vi "CGTdaq dev V4.vi"() -> ()   [LabVIEW 2023]
panel:
  in  "?":bool
  in  "?":bool
  in  "Path":path
  in  "File extension":string
  in  "Filename":string
  out "?":timestamp
  in  "stop":bool
  in  "?":bool
  in  "?":bool
  in  "?":T1(tab)
  in  "Plotted Port":dbl
  out "?":dbl(graph)
  in  "Input Val":dbl
  out "LabJack Error":errorcluster
  out "Error Message":string
  in  "Scan Rate (Hz)":dbl=10.0 format="%.3f"
  out "# Scans Read":i32
  out "Actual Scan Rate (Hz)":dbl format="%.3f"
  out "UD Backlog [%]":dbl format="%.2f"
  in  "Scans To Read Per Iteration":dbl=1.0 format="%.3f"
  out "Comm Backlog [%]":dbl format="%.2f"
  in  "Delay [ms]":u32
  in  "Res Index":dbl
  out "Full filepath":string
  out "A5 Scaled":dbl(graph)
  out "A4 Scaled":dbl(graph)
  out "A3 Scaled":dbl(graph)
  out "A2 Scaled":dbl(graph)
  out "A1 Scaled":dbl(graph)
  out "A0 Scaled":dbl(graph)
  out "A1":dbl
  out "A1_Voltage":dbl
  out "A1_Instrumentlabel":string
  out "A2 X1 2":dbl caption="A0 X1"
  out "A2 X2 2":dbl caption="A0 X2"
  out "A2 X3 2":dbl caption="A0 X3"
  out "A2 B 2":dbl caption="A0 B"
  out "A2 scaled 2":dbl caption="A0 scaled"
  out "A1_Instrumentlabel 2":string
  out "A1_Voltage 3":dbl
  out "A1 2":dbl
  out "A2 X1 3":dbl caption="A0 X1"
  out "A2 X2 3":dbl caption="A0 X2"
  out "A2 X3 3":dbl caption="A0 X3"
  out "A2 B 3":dbl caption="A0 B"
  out "A2 scaled 3":dbl caption="A0 scaled"
  out "A2 scaled 4":dbl caption="A0 scaled"
  out "A1_Instrumentlabel 3":string
  out "A2 X1 4":dbl caption="A0 X1"
  out "A2 X2 4":dbl caption="A0 X2"
  out "A2 X3 4":dbl caption="A0 X3"
  out "A2 B 4":dbl caption="A0 B"
  out "A1_Voltage 2":dbl
  out "A1 3":dbl
  out "A1_Instrumentlabel 4":string
  out "A1 4":dbl
  out "A1_Voltage 4":dbl
  out "A2 scaled 5":dbl caption="A0 scaled"
  out "A2 X2 5":dbl caption="A0 X2"
  out "A2 X3 5":dbl caption="A0 X3"
  out "A2 B 5":dbl caption="A0 B"
  out "A2 X1 5":dbl caption="A0 X1"
  out "A1_Instrumentlabel 5":string
  out "A1 5":dbl
  out "A1_Voltage 5":dbl
  out "A2 X1 6":dbl caption="A0 X1"
  out "A2 X2 6":dbl caption="A0 X2"
  out "A2 X3 6":dbl caption="A0 X3"
  out "A2 B 6":dbl caption="A0 B"
  out "A2 scaled 6":dbl caption="A0 scaled"
  out "A1_Instrumentlabel 6":string
  out "A1 6":dbl
  out "A1_Voltage 6":dbl
  out "A2 X1 7":dbl caption="A0 X1"
  out "A2 X2 7":dbl caption="A0 X2"
  out "A2 X3 7":dbl caption="A0 X3"
  out "A2 B 7":dbl caption="A0 B"
  out "A2 scaled 7":dbl caption="A0 scaled"
  out "A1_Instrumentlabel 7":string
  out "A1 7":dbl
  out "A1_Voltage 7":dbl
  out "A2 scaled 8":dbl caption="A0 scaled"
  out "A2 X2 8":dbl caption="A0 X2"
  out "A2 X1 8":dbl caption="A0 X1"
  out "A2 B 8":dbl caption="A0 B"
  out "A2 X3 8":dbl caption="A0 X3"
  out "A1_Instrumentlabel 8":string
  out "A1 8":dbl
  out "A1_Voltage 8":dbl
  out "A2 X1 9":dbl caption="A0 X1"
  out "A2 X2 9":dbl caption="A0 X2"
  out "A2 X3 9":dbl caption="A0 X3"
  out "A2 B 9":dbl caption="A0 B"
  out "A2 scaled 9":dbl caption="A0 scaled"
  out "A1_Instrumentlabel 9":string
  out "A1 9":dbl
  out "A1_Voltage 9":dbl
  out "A2 X1 10":dbl caption="A0 X1"
  out "A2 X2 10":dbl caption="A0 X2"
  out "A2 X3 10":dbl caption="A0 X3"
  out "A2 B 10":dbl caption="A0 B"
  out "A2 scaled 10":dbl caption="A0 scaled"
  # "."
  # "Analog Port"
  # "Voltage In"
  # "X3"
  # "X1"
  # "B"
  # "Instrument name"
  # "X2"
  # "Scaled Value"
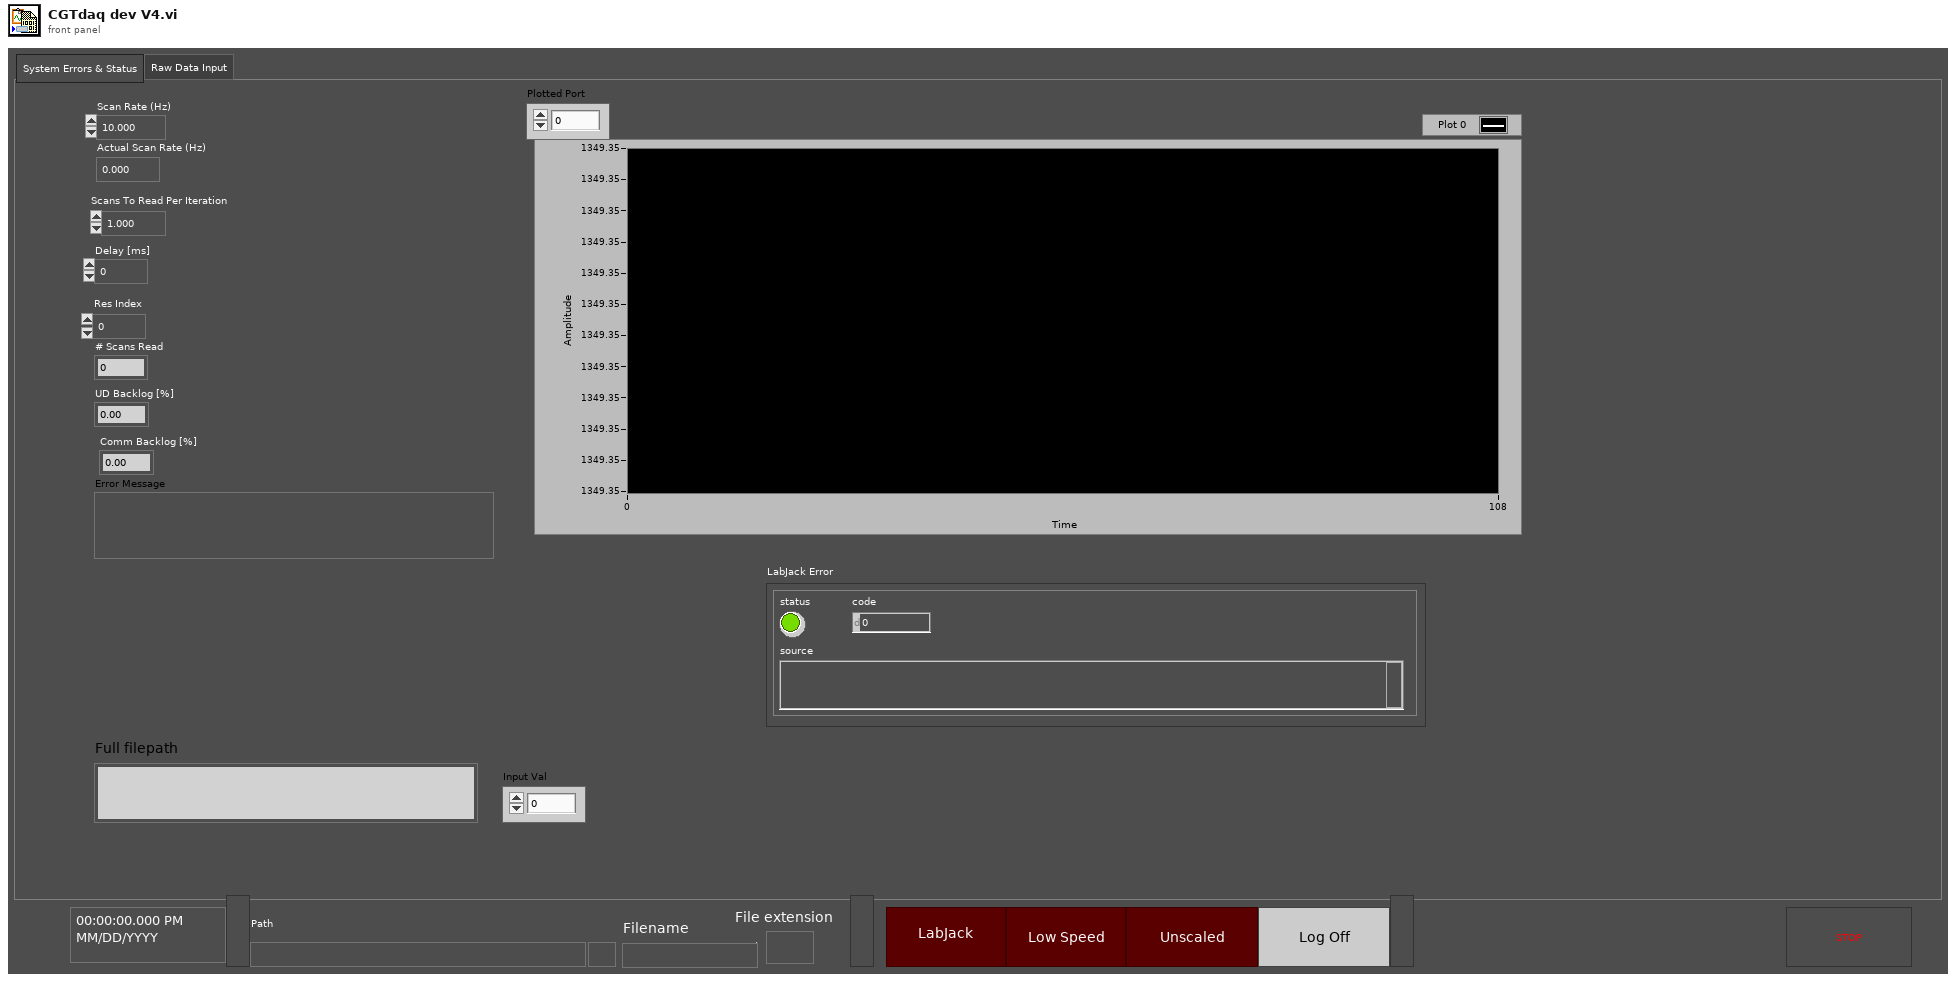
[diagram p1: front panel]
types:
  T1 = enum32{"System Errors & Status", "Raw Data Input"}
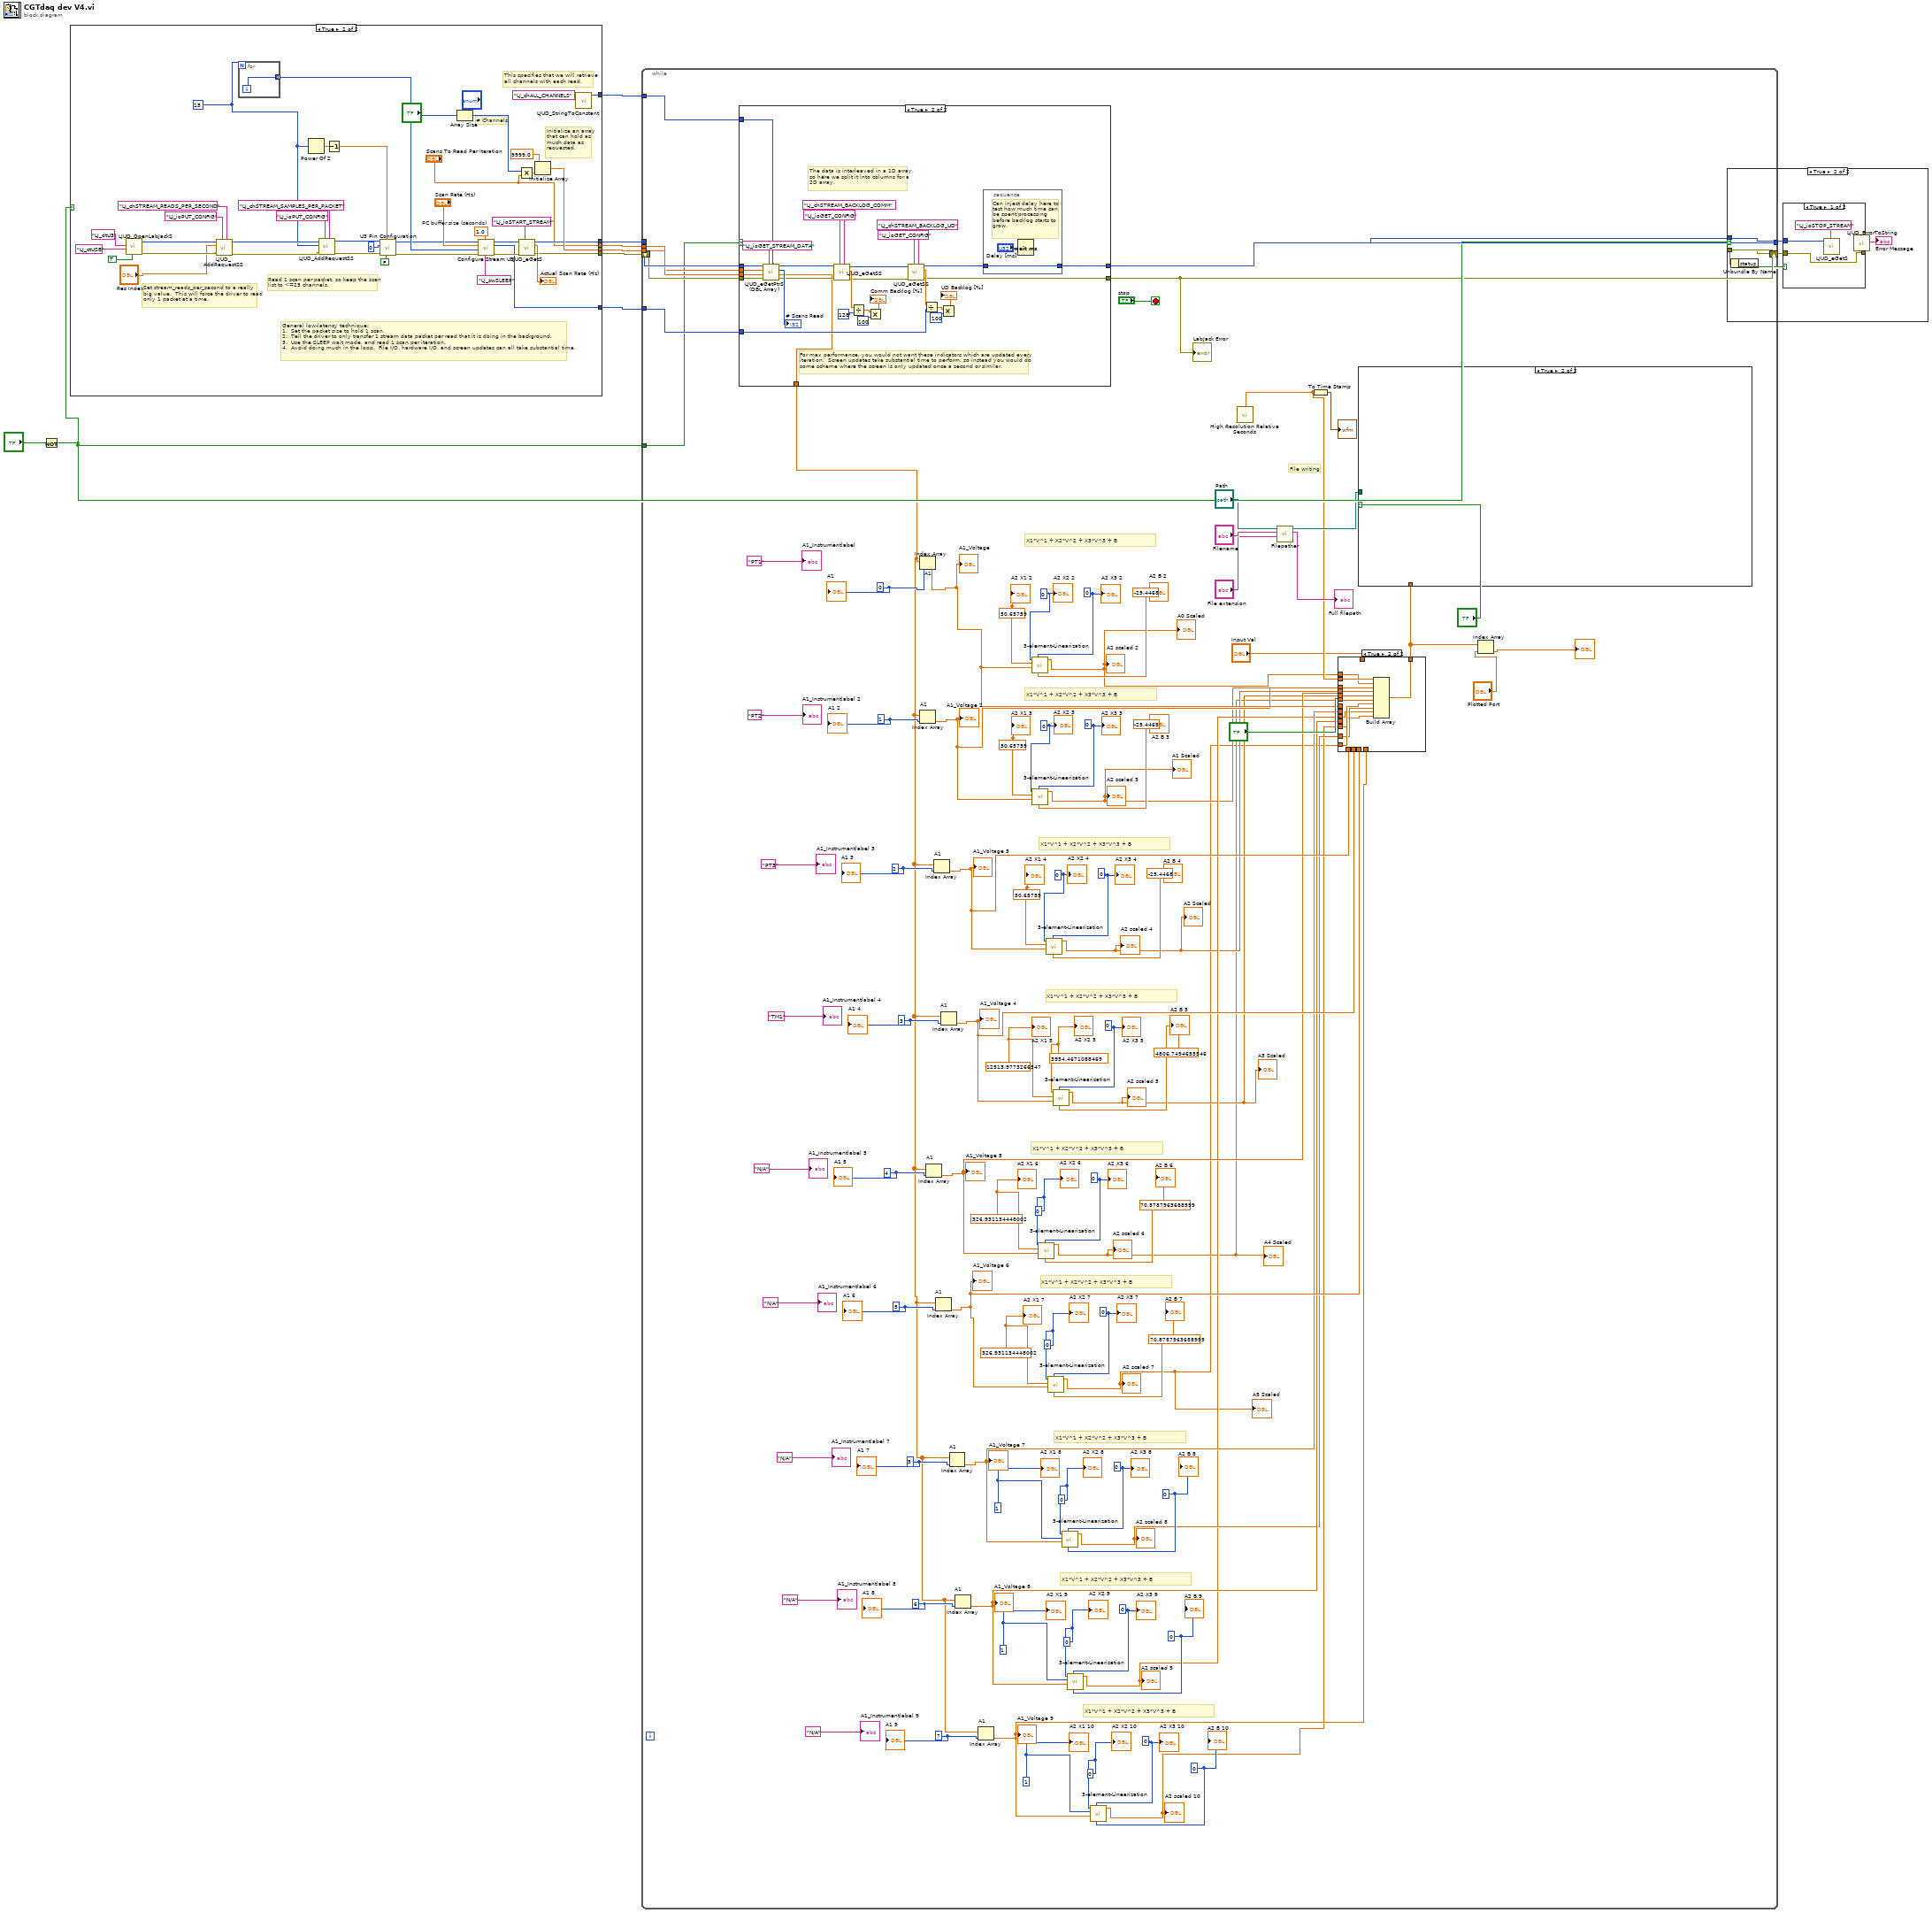
[diagram p0: block diagram]
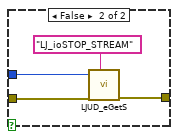
[diagram p3: hidden frame]
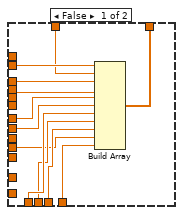
[diagram p5: hidden frame]
diagram:
  n1 = Not(x="?") -> (.not. x?=w2:bool)
  n2 = case shown="True" w2 {
    tunnel: [_ w44] -> w10
    tunnel: [_ w40] -> w8
    tunnel: [_ w38] -> w7
    tunnel: [_ w37] -> w5
    tunnel: [_ w34] -> w4
    tunnel: [_ "Scans To Read Per Iteration"] -> w3
    frame False {
    }
    frame True {
      w11 = 15
      w22 = 1.0  # PC buffer size (seconds)
      # "General low-latency technique:\n1.  Set the packet size to hold 1 scan.\n2.  Tell the driver to only transfer 1 stream data packet per read that it is doing in the background.\n3.  Use the SLEEP wait mode, and read 1 scan per iteration.\n4.  Avoid doing much in the loop.  File I/O, hardware I/O, and screen updates can all take substantial time."
      # "Set stream_reads_per_second to a really\nbig value.  This will force the driver to read\nonly 1 packet at a time."
      # "Read 1 scan per packet, so keep the scan\nlist to <=25 channels."
      # "Initialize an array\nthat can hold as\nmuch data as\nrequested."
      # "# Channels"
      # "This specifies that we will retrieve\nall channels with each read."
      n3 = call <vilib>:"LJUD_OpenLabJackS.vi"("FirstFound"=TRUE, "ConnectionType"="LJ_ctUSB", "DeviceType"="LJ_dtU3") -> ("error out"=w25:errorcluster, "Handle"=w27:i32)  [unwired: 6 in, 1 out]
      n4 = call <vilib>:"LJUD_AddRequestSS.vi"("Channel"="LJ_chSTREAM_READS_PER_SECOND" ("IOType"), "IOType"="LJ_ioPUT_CONFIG", "error in"=w25, "Value"="Res Index", "Handle In"=w27) -> ("error out"=w24:errorcluster, "Handle Out"=w26:i32)  [unwired: 5 in]
      n5 = for {
        N: w11 -> [_]
        tunnel: [w50] -> w21 mode=indexing
        i -> [w50]
      }
      n6 = Power Of 2(x=w11) -> (2^x=w14:dbl)
      n7 = call <vilib>:"LJUD_AddRequestSS.vi"("Channel"="LJ_chSTREAM_SAMPLES_PER_PACKET" ("IOType"), "IOType"="LJ_ioPUT_CONFIG", "error in"=w24, "Value"=w11, "Handle In"=w26) -> ("error out"=w20:errorcluster, "Handle Out"=w18:i32)  [unwired: 5 in]
      n8 = Decrement(x=w14) -> (x-1=w13:dbl)
      n9 = call <vilib>:"U3 Pin Configuration.vi"("Enable Counter0"=FALSE, "FIO/EIO Analog Enable"=w13, "error in"=w20, "Number of Timers Enabled"=u8 0, "Handle In"=w18) -> ("error out"=w19:errorcluster, "Handle Out"=w17:i32)  [unwired: 5 in]
      n10 = Array Size(array=w21) -> (size(s)=w43:i32)
      n11 = call <vilib>:"Configure Stream U3.vi"("Wait Mode"="LJ_swSLEEP" ("Wait Mode (2)"), "PC buffer size (seconds)"=w22, "error in"=w19, "Scan List (+)"=w21, "Scan Rate (Hz)"="Scan Rate (Hz)", "Handle In"=w17) -> ("error out"=w47:errorcluster, "PC buffer size (samples)"=w34:i32, "Handle Out"=w48:i32)  [unwired: 3 in]
      n12 = Multiply(x=w43, y="Scans To Read Per Iteration") -> (x*y=w46:dbl)
      n13 = call <vilib>:"LJUD_eGetS.vi"("IOType"="LJ_ioSTART_STREAM", "error in"=w47, "Handle In"=w48) -> ("error out"=w37:errorcluster, "Value Read"=→"Actual Scan Rate (Hz)":dbl, "Handle Out"=w40:i32)  [unwired: 6 in]
      n14 = Initialize Array(9999.0, w46) -> (w44:dbl[])
      n15 = call <vilib>:"LJUD_StringToConstant.vi"("String"="LJ_chALL_CHANNELS") -> ("Constant Number"=w38:i32)  [unwired: 9 in, 1 out]
    }
  }
  n16 = while {
    tunnel: w4 -> [w141]
    shift-left: w5 -> [w142]
    shift-right: [w82] -> w6
    tunnel: w7 -> [w143]
    tunnel: [w140] -> w9
    tunnel: w10 -> [w145]
    tunnel: w3 -> [w144]
    tunnel: w8 -> [w146]
    tunnel: w2 -> [w139]
    stop <- "stop" stop-if-true
    w84 = 0
    w87 = 0
    w86 = 0
    w85 = 1
    w89 = 7
    w90 = 0
    w93 = 0
    w92 = 0
    w91 = 1
    w95 = 6
    w96 = 0
    w99 = 0
    w98 = 0
    w97 = 1
    w101 = 5
    w102 = 70.8787963688999
    w105 = 0
    w104 = 0
    w103 = 326.931134448002
    w107 = 5
    w108 = 70.8787963688999
    w111 = 0
    w110 = 0
    w109 = 326.931134448002
    w113 = 4
    w114 = 4806.7494655546
    w117 = 0
    w116 = 3954.4671088469
    w115 = 12513.9773266547
    w119 = 3
    w120 = -25.4468
    w123 = 0
    w122 = 0
    w121 = 50.65759
    w125 = 2
    w126 = -25.4468
    w129 = 0
    w128 = 0
    w127 = 50.65759
    w131 = 1
    w132 = -25.4468
    w135 = 0
    w134 = 0
    w133 = 50.65759
    w137 = 0
    # "File writing"
    # "X1*V^1 + X2*V^2 + X3*V^3 + B"
    # "X1*V^1 + X2*V^2 + X3*V^3 + B"
    # "X1*V^1 + X2*V^2 + X3*V^3 + B"
    # "X1*V^1 + X2*V^2 + X3*V^3 + B"
    # "X1*V^1 + X2*V^2 + X3*V^3 + B"
    # "X1*V^1 + X2*V^2 + X3*V^3 + B"
    # "X1*V^1 + X2*V^2 + X3*V^3 + B"
    # "X1*V^1 + X2*V^2 + X3*V^3 + B"
    # "X1*V^1 + X2*V^2 + X3*V^3 + B"
    n17 = case shown="True" w139 {
      tunnel: w146 -> [_ w198]
      tunnel: w145 -> [_ w196]
      tunnel: w144 -> [_ w195]
      tunnel: w143 -> [_ w194]
      tunnel: w142 -> [_ w192]
      tunnel: [_ w185] -> w82
      tunnel: w141 -> [_ w184]
      tunnel: [_ w182] -> w140
      tunnel: [_ w170] -> w83
      frame False {
      }
      frame True {
        # "For max performance, you would not want these indicators which are updated every\niteration.  Screen updates take substantial time to perform, so instead you would do\nsome scheme where the screen is only updated once a second or similar."
        # "The data is interleaved in a 1D array,\nso here we split it into columns for a\n2D array."
        n18 = call <vilib>:"LJUD_eGetPtrS (DBL Array).vi"("Channel"=w194, "IOType"="LJ_ioGET_STREAM_DATA", "error in"=w192, "DBL Array Write"=w196, "Value"=w195, "Handle In"=w198) -> ("error out"=w173:errorcluster, "DBL Array Read"=w170:dbl[], "Value"=→"# Scans Read":i32, "Handle Out"=w172:i32)  [unwired: 2 in]
        n19 = call <vilib>:"LJUD_eGetSS.vi"("Channel"="LJ_chSTREAM_BACKLOG_COMM", "IOType"="LJ_ioGET_CONFIG", "error in"=w173, "Handle In"=w172) -> ("error out"=w174:errorcluster, "Value Read"=w181:dbl, "Handle Out"=w175:i32)  [unwired: 5 in]
        n20 = Divide(x=w181, y=128) -> (x/y=w178:dbl)
        n21 = Multiply(x=w178, y=100) -> (x*y=→"Comm Backlog [%]":dbl)
        n22 = call <vilib>:"LJUD_eGetSS.vi"("Channel"="LJ_chSTREAM_BACKLOG_UD", "IOType"="LJ_ioGET_CONFIG", "error in"=w174, "Handle In"=w175) -> ("error out"=w185:errorcluster, "Value Read"=w187:dbl, "Handle Out"=w183:i32)  [unwired: 5 in]
        n23 = Divide(x=w187, y=w184) -> (x/y=w188:dbl)
        n24 = Multiply(x=w188, y=100) -> (x*y=→"UD Backlog [%]":dbl)
        n25 = stacked-sequence {
          tunnel: w183 -> [w200]
          tunnel: [w200] -> w182
          frame #0 {
            # "Can inject delay here to\ntest how much time can\nbe spent processing\nbefore backlog starts to\ngrow."
            n26 = Wait (ms)(milliseconds to wait="Delay [ms]") -> ()  [unwired: 1 out]
          }
        }
      }
    }
    "LabJack Error" <- w82
    n27 = Index Array "A1"(array=w83, index=w137) -> (element=w72:dbl)
    "A1_Voltage" <- w72
    n28 = Index Array "A1"(array=w83, index=w131) -> (element=w71:dbl)
    "A1_Voltage 2" <- w71
    n29 = Index Array "A1"(array=w83, index=w113) -> (element=w68:dbl)
    "A1_Voltage 5" <- w68
    n30 = Index Array "A1"(array=w83, index=w125) -> (element=w70:dbl)
    "A1_Voltage 3" <- w70
    n31 = Index Array "A1"(array=w83, index=w107) -> (element=w67:dbl)
    "A1_Voltage 6" <- w67
    n32 = Index Array "A1"(array=w83, index=w119) -> (element=w69:dbl)
    "A1_Voltage 4" <- w69
    n33 = Index Array "A1"(array=w83, index=w101) -> (element=w66:dbl)
    "A1_Voltage 7" <- w66
    n34 = Index Array "A1"(array=w83, index=w95) -> (element=w64:dbl)
    "A1_Voltage 8" <- w64
    n35 = Index Array "A1"(array=w83, index=w89) -> (element=w63:dbl)
    "A1_Voltage 9" <- w63
    n36 = call "3-element-Linearization.vi"("B"=w132, "C3"=w135, "Voltage in"=w72, "C1"=w133, "C2"=w134) -> ("Scaled value"=w56:dbl)  [unwired: 6 in]
    "A2 scaled 2" <- w56
    "A0 Scaled" <- w56
    n37 = call "3-element-Linearization.vi"("B"=w126, "C3"=w129, "Voltage in"=w71, "C1"=w127, "C2"=w128) -> ("Scaled value"=w55:dbl)  [unwired: 6 in]
    "A2 scaled 3" <- w55
    "A1 Scaled" <- w55
    n38 = call "3-element-Linearization.vi"("B"=w108, "C3"=w111, "Voltage in"=w68, "C1"=w109, "C2"=w110) -> ("Scaled value"=w52:dbl)  [unwired: 6 in]
    "A2 scaled 6" <- w52
    "A4 Scaled" <- w52
    n39 = call "3-element-Linearization.vi"("B"=w120, "C3"=w123, "Voltage in"=w70, "C1"=w121, "C2"=w122) -> ("Scaled value"=w54:dbl)  [unwired: 6 in]
    "A2 scaled 4" <- w54
    "A2 Scaled" <- w54
    n40 = call "3-element-Linearization.vi"("B"=w102, "C3"=w105, "Voltage in"=w67, "C1"=w103, "C2"=w104) -> ("Scaled value"=w51:dbl)  [unwired: 6 in]
    "A2 scaled 7" <- w51
    "A5 Scaled" <- w51
    n41 = call "3-element-Linearization.vi"("B"=w114, "C3"=w117, "Voltage in"=w69, "C1"=w115, "C2"=w116) -> ("Scaled value"=w53:dbl)  [unwired: 6 in]
    "A2 scaled 5" <- w53
    "A3 Scaled" <- w53
    n42 = call "3-element-Linearization.vi"("B"=w96, "C3"=w99, "Voltage in"=w66, "C1"=w97, "C2"=w98) -> ("Scaled value"=w62:dbl)  [unwired: 6 in]
    "A2 scaled 8" <- w62
    n43 = call "3-element-Linearization.vi"("B"=w90, "C3"=w93, "Voltage in"=w64, "C1"=w91, "C2"=w92) -> ("Scaled value"=w61:dbl)  [unwired: 6 in]
    "A2 scaled 9" <- w61
    n44 = call "3-element-Linearization.vi"("B"=w84, "C3"=w87, "Voltage in"=w63, "C1"=w85, "C2"=w86) -> ("Scaled value"=w60:dbl)  [unwired: 6 in]
    "A2 scaled 10" <- w60
    n45 = call <vilib>:"High Resolution Relative Seconds.vi"() -> ("relative seconds"=w74:dbl)
    n46 = call "Filepather.vi"("File extension"="File extension", "Filename"="Filename", "Path in"="Path") -> ("Full filepath"=→"Full filepath":string, "Path out"=w75:path)  [unwired: 7 in]
    n47 = To Time Stamp(1:w74) -> (0:→"?":timestamp)
    n48 = case shown="True" "?" {
      tunnel: w74 -> [w158 w169]
      tunnel: w72 -> [w154 _]
      tunnel: w71 -> [w156 _]
      tunnel: w70 -> [w152 _]
      tunnel: w69 -> [w151 _]
      tunnel: w68 -> [w155 _]
      tunnel: w67 -> [w150 _]
      tunnel: w66 -> [w153 _]
      tunnel: "Input Val" -> [w157 _]
      tunnel: w64 -> [w149 _]
      tunnel: w63 -> [w148 _]
      tunnel: [w147 w168] -> w59
      tunnel: w56 -> [_ w167]
      tunnel: w55 -> [_ w166]
      tunnel: w54 -> [_ w165]
      tunnel: w53 -> [_ w164]
      tunnel: w52 -> [_ w163]
      tunnel: w51 -> [_ w162]
      tunnel: w62 -> [_ w161]
      tunnel: w61 -> [_ w160]
      tunnel: w60 -> [_ w159]
      frame False {
        n49 = Build Array(w158, w157, w156, w155, w154, w153, w152, w151, w150, w149, w148) -> (w147:dbl[])
      }
      frame True {
        n50 = Build Array(w169, w167, w166, w165, w164, w163, w162, w161, w160, w159) -> (w168:dbl[])
      }
    }
    n51 = case shown="True" "?" {
      tunnel: w75 -> [_ _]
      tunnel: w59 -> [_ _]
      frame False {
      }
      frame True {
      }
    }
    n52 = Index Array(array=w59, index="Plotted Port") -> (element=→"?":dbl)
    "A1" <- w137
    "A1_Instrumentlabel" <- "PT1"
    "A2 X1 2" <- w133
    "A2 X2 2" <- w134
    "A2 X3 2" <- w135
    "A2 B 2" <- w132
    "A1 2" <- w131
    "A1_Instrumentlabel 2" <- "PT2"
    "A2 X1 3" <- w127
    "A2 X2 3" <- w128
    "A2 X3 3" <- w129
    "A2 B 3" <- w126
    "A1 3" <- w125
    "A1_Instrumentlabel 3" <- "PT3"
    "A2 X1 4" <- w121
    "A2 X2 4" <- w122
    "A2 X3 4" <- w123
    "A2 B 4" <- w120
    "A1 4" <- w119
    "A1_Instrumentlabel 4" <- "TM1"
    "A2 X1 5" <- w115
    "A2 X2 5" <- w116
    "A2 X3 5" <- w117
    "A2 B 5" <- w114
    "A1 5" <- w113
    "A1_Instrumentlabel 5" <- "N/A"
    "A2 X1 6" <- w109
    "A2 X2 6" <- w110
    "A2 X3 6" <- w111
    "A2 B 6" <- w108
    "A1 6" <- w107
    "A1_Instrumentlabel 6" <- "N/A"
    "A2 X1 7" <- w103
    "A2 X2 7" <- w104
    "A2 X3 7" <- w105
    "A2 B 7" <- w102
    "A1 7" <- w101
    "A1_Instrumentlabel 7" <- "N/A"
    "A2 X1 8" <- w97
    "A2 X2 8" <- w98
    "A2 X3 8" <- w99
    "A2 B 8" <- w96
    "A1 8" <- w95
    "A1_Instrumentlabel 8" <- "N/A"
    "A2 X1 9" <- w91
    "A2 X2 9" <- w92
    "A2 X3 9" <- w93
    "A2 B 9" <- w90
    "A1 9" <- w89
    "A1_Instrumentlabel 9" <- "N/A"
    "A2 X1 10" <- w85
    "A2 X2 10" <- w86
    "A2 X3 10" <- w87
    "A2 B 10" <- w84
  }
  n53 = case shown="True" w2 {
    tunnel: w9 -> [_ w204]
    tunnel: w6 -> [_ w201]
    frame False {
    }
    frame True {
      n54 = Unbundle By Name(w201) -> ("status"=w202:bool)
      n55 = case shown="True" w202 {
        tunnel: w204 -> [w207 w211]
        tunnel: [w206 w210] -> w203
        tunnel: w201 -> [w206 w209]
        frame True {
          n56 = call <vilib>:"LJUD_eGetS.vi"("IOType"="LJ_ioSTOP_STREAM", "Handle In"=w207) -> ()  [unwired: 7 in, 3 out]
        }
        frame False {
          n57 = call <vilib>:"LJUD_eGetS.vi"("IOType"="LJ_ioSTOP_STREAM", "error in"=w209, "Handle In"=w211) -> ("error out"=w210:errorcluster)  [unwired: 6 in, 2 out]
        }
      }
      n58 = call <vilib>:"LJUD_ErrorToString.vi"("error in"=w203) -> ("String"=→"Error Message":string)  [unwired: 10 in]
    }
  }
